vi "Camera Calculator.vi"() -> ()   [LabVIEW 2015]
uses:
  <vilib>/gmath/NI_Gmath.lvlib
panel:
  out "Answer":dbl format="%0.2f"
  in  "plus":bool
  in  "one":bool
  out "one":i32
  in  "stop":bool
  out "Equation":string
  out "Plus":i32
  in  "Stop (F)":bool
  out "Image Out":T1(plugin-control)
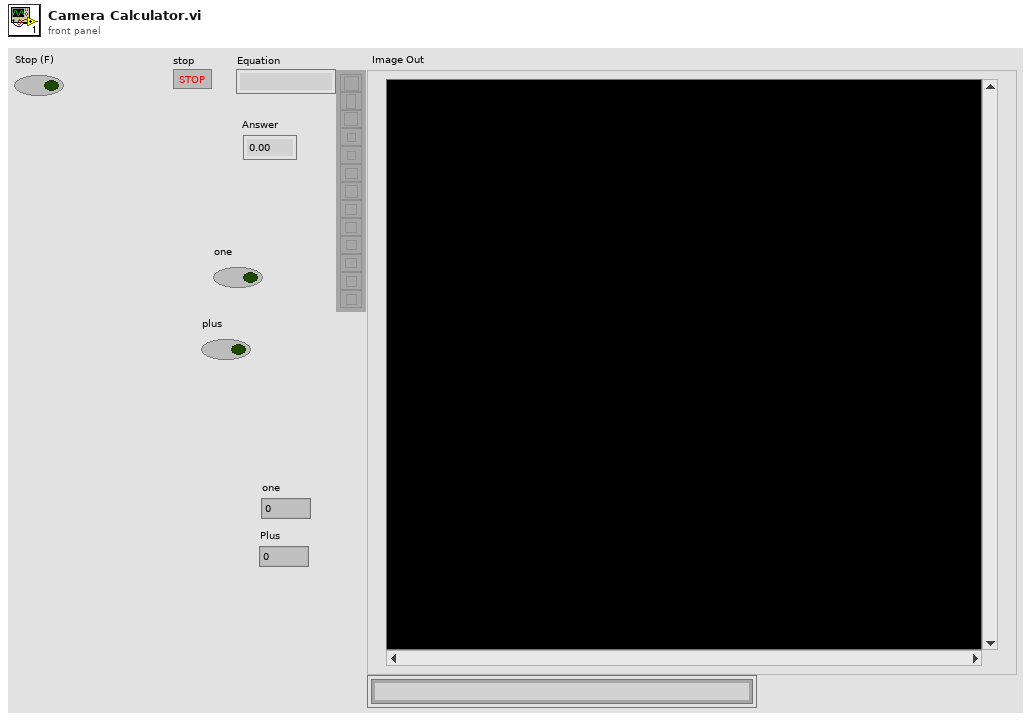
[diagram p1: front panel]
types:
  T1 = typedef "IMAQ Image.ctl" = refnum<image>
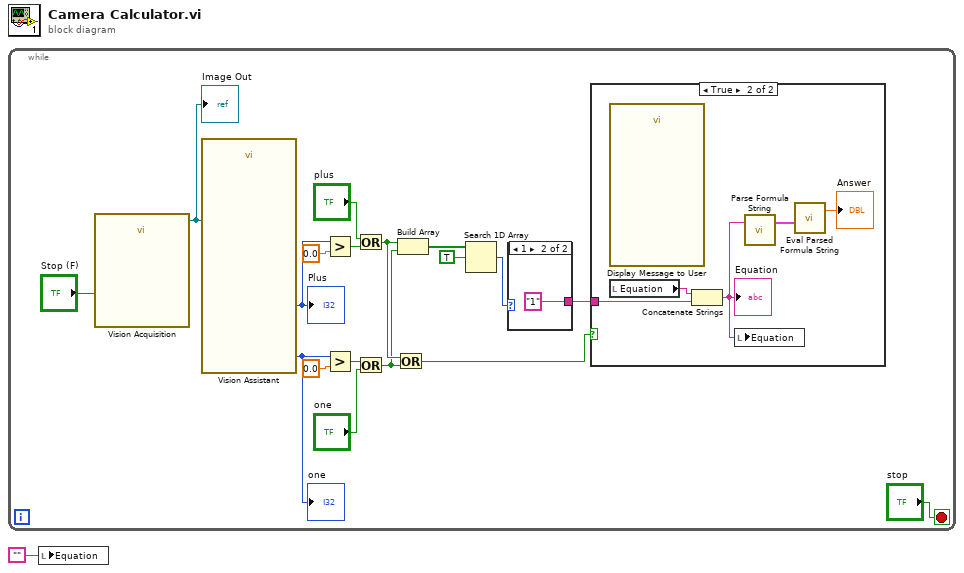
[diagram p0: block diagram]
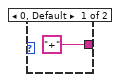
[diagram p3: hidden frame]
diagram:
  n1 = while {
    stop <- "stop" stop-if-true
    n2 = call "Vision Acquisition"("Stop (F)"="Stop (F)") -> ("Image Out"=w18:T1)  [unwired: 24 in, 2 out]
    "Image Out" <- w18
    n3 = call "Vision Assistant"("Image In"=w18) -> ("Number of Matches (Geometric Matching 1)"=w16:i32, "Number of Matches (Geometric Matching 2)"=w9:i32)  [unwired: 21 in, 4 out]
    "Plus" <- w16
    "one" <- w9
    n4 = Greater?(x=w16, y=0.0) -> (0:w6:bool)
    n5 = Greater?(x=w9, y=0.0) -> (0:w4:bool)
    n6 = Or(x="plus", y=w6) -> (x .or. y?=w5:bool)
    n7 = Or(x=w4, y="one") -> (x .or. y?=w2:bool)
    n8 = Or(x=w5, y=w2) -> (x .or. y?=w8:bool)
    n9 = Build Array(w5, w2) -> (w13:bool[])
    n10 = Search 1D Array(1D array=w13, element=TRUE) -> (index of element=w14:i32)  [unwired: 1 in]
    n11 = case shown="1" w14 {
      tunnel: ["+" "1"] -> w11
      frame 0, Default {
      }
      frame 1 {
      }
    }
    n12 = case shown="True" w8 {
      tunnel: w11 -> [_ w24]
      frame False {
      }
      frame True {
        n13 = call "Display Message to User"() -> ()  [unwired: 10 in, 2 out]
        n14 = local read "Equation"() -> (w23:string)
        n15 = Concatenate Strings(w23, w24) -> (w20:string)
        "Equation" <- w20
        n16 = local write "Equation"(w20) -> ()
        n17 = call <vilib>:"Parse Formula String.vi"("formula"=w20) -> ("Parsed Formula"=w21:cluster{"Table":i32[][], "Y Values":dbl[]})  [unwired: 1 in, 1 out]
        n18 = call <vilib>:"Eval Parsed Formula String.vi"("Parsed Formula"=w21) -> ("y value"=→"Answer":dbl)  [unwired: 3 in, 1 out]
      }
    }
  }
  n19 = local write "Equation"("") -> ()
